vi "Drawbridge Controller.vi"(8 "error in":errorcluster) -> ()   [LabVIEW 2015]
doc: "This VI executes continuously carrying out the current operation and responding to updates or new operations. It will often contain the timing or control code that is difficult to place directly in TeleOp. This VI generally opens all sensors and motors and isolates the rest of the robot code from knowing how the operations are carried out."
uses:
  Drawbridge Setpoints.ctl
  Drawbridge Operations.ctl
  Framework/Motor Ref Names Type Def.ctl
panel:
  out "Current\nCmd":string
  # "Tip: It may be helpful to observe inputs and sensor values.\nYou may also want to display tuning or debugging controls."
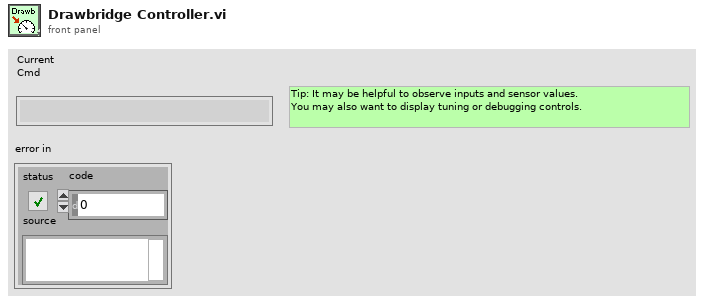
[diagram p1: front panel]
types:
  T1 = typedef "Motor Ref Names Type Def.ctl" = enum16{"Angular Motor"}
  T2 = typedef "Drawbridge Setpoints.ctl" = cluster{"Operation":T3, "Setpoint":dbl, "Duration":dbl}
  T3 = typedef "Drawbridge Operations.ctl" = enum16{"Reserve", "Read Current", "Immediate", "Open"}
  T4 = typedef "Command Status Info.ctl" = cluster{"Name":string, "Status":T5, "notifier out":T6}
  T5 = typedef "Completion Status.ctl" = enum16{"Successful", "Aborted", "Incomplete"}
  T6 = typedef "Completion Notifier.ctl" = refnum<notifier>
  T7 = cluster{"Default Command":T2, "Command Timing":cluster{"Start Time (ms)":u32, "Iterations":i32}, "Command Arguments":cluster{"Command Info":T4, "Description":string, "Default Command":T2, "notifier out":refnum<notifier>, "Subsystem Name":string}}
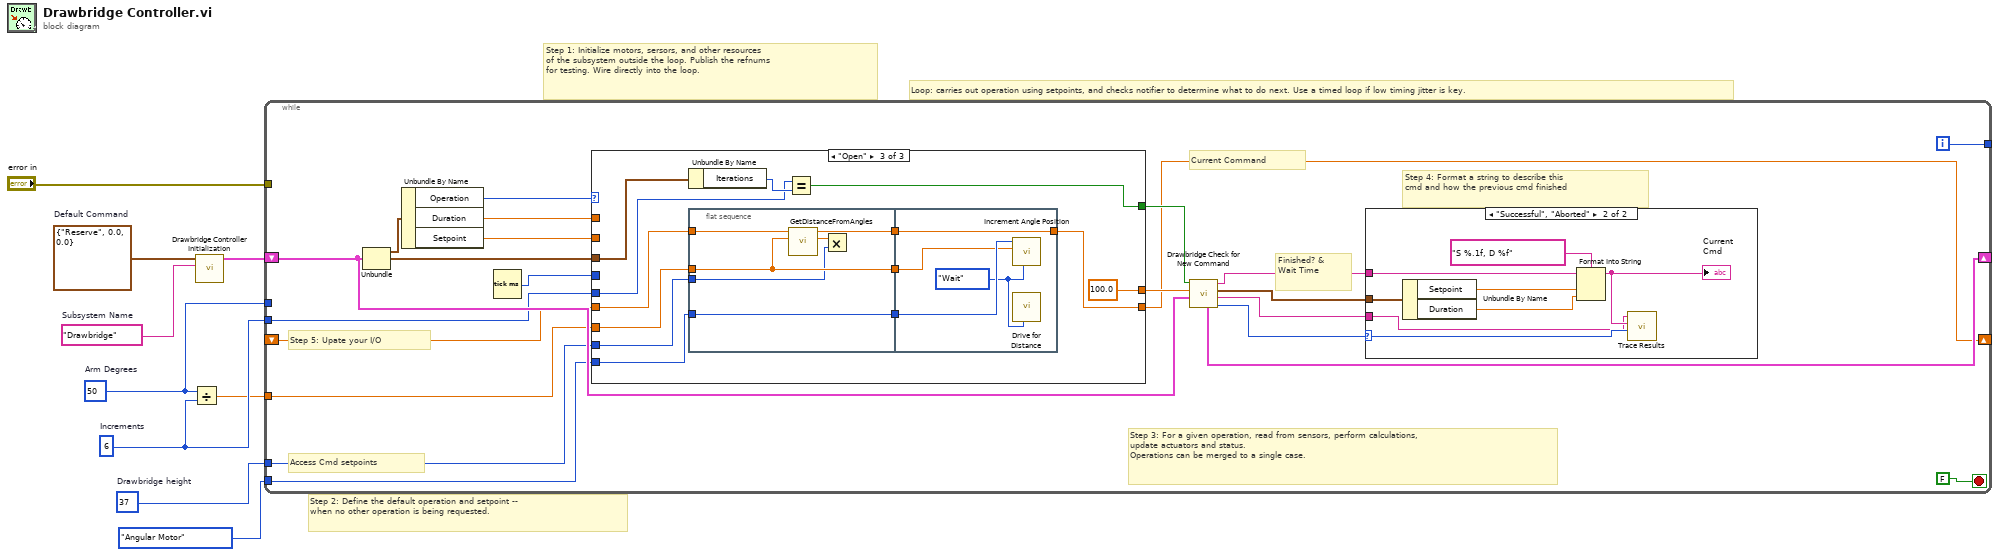
[diagram p0: block diagram]
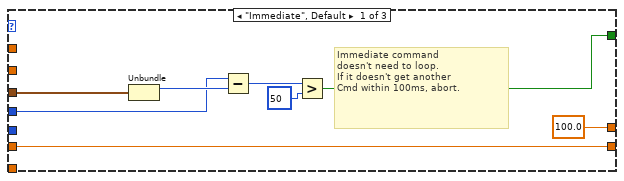
[diagram p3: hidden frame]
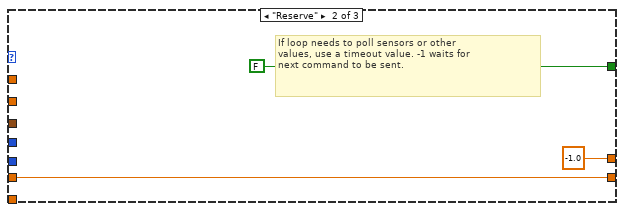
[diagram p4: hidden frame]
diagram:
  w1 = 37  # Drawbridge height
  w4 = 50  # Arm Degrees
  w3 = 6  # Increments
  w6 = T2 {"Operation"=enum."Reserve", "Setpoint"=0.0, "Duration"=0.0}  # Default Command
  w7 = "Drawbridge"  # Subsystem Name
  # "Step 2: Define the default operation and setpoint --\nwhen no other operation is being requested."
  # "Step 1: Initialize motors, sersors, and other resources\nof the subsystem outside the loop. Publish the refnums\nfor testing. Wire directly into the loop."
  # "Loop: carries out operation using setpoints, and checks notifier to determine what to do next. Use a timed loop if low timing jitter is key."
  n1 = Divide(x=w4, y=w3) -> (x/y=w2:dbl)
  n2 = call "Drawbridge Controller Initialization.vi"("Subsystem Name"=w7, "Default Command"=w6) -> ("Command Info"=w8:T7)  [unwired: 9 in]
  n3 = while {
    shift-right: [w22] -> _
    shift-left: w8 -> [w23]
    tunnel: [w30] -> _
    tunnel: "error in" -> [_]
    shift-right: [w14] -> _
    shift-left: _ -> [w15]
    tunnel: w3 -> [w13]
    tunnel: w4 -> [_]
    tunnel: Motor_Ref_Names_Type_Def."Angular Motor" ("Motor Ref Names") -> [w12]
    tunnel: w2 -> [w11]
    tunnel: w1 -> [w10]
    i -> [w30]
    stop <- FALSE stop-if-true
    # "Step 5: Upate your I/O"
    # "Step 4: Format a string to describe this\ncmd and how the previous cmd finished"
    # "Current Command"
    # "Access Cmd setpoints"
    # "Finished? &\nWait Time"
    # "Step 3: For a given operation, read from sensors, perform calculations,\nupdate actuators and status.\nOperations can be merged to a single case."
    n4 = Unbundle(w23) -> ("Default Command"=w29:T2, "Command Timing"=w25:cluster{"Start Time (ms)":u32, "Iterations":i32})  [unwired: 1 out]
    n5 = Unbundle By Name(w29) -> ("Operation"=w28:T3, "Duration"=w27:dbl, "Setpoint"=w24:dbl)
    n6 = Tick Count (ms)() -> (millisecond timer value=w26:u32)
    n7 = case shown="\"Open\"" w28 {
      tunnel: [100.0 -1.0 100.0] -> w20
      tunnel: [w41 FALSE ("ignore previous (F)") w55] -> w21
      tunnel: w25 -> [w43 _ w58]
      tunnel: w27 -> [_ _ _]
      tunnel: w26 -> [w42 _ _]
      tunnel: w24 -> [_ _ _]
      tunnel: w15 -> [w40 w48 w62]
      tunnel: w11 -> [_ _ w61]
      tunnel: [w40 w48 w59] -> w14
      tunnel: w13 -> [_ _ w56]
      tunnel: w12 -> [_ _ w53]
      tunnel: w10 -> [_ _ w51]
      frame "Immediate", Default {
        # "Immediate command\ndoesn't need to loop.\nIf it doesn't get another\nCmd within 100ms, abort."
        n8 = Unbundle(w43) -> ("Start Time (ms)"=w46:u32)  [unwired: 1 out]
        n9 = Subtract(x=w42, y=w46) -> (x-y=w45:u32)
        n10 = Greater?(x=w45, y=u8 50 ("Left Motor")) -> (0:w41:bool)
      }
      frame "Reserve" {
        # "If loop needs to poll sensors or other\nvalues, use a timeout value. -1 waits for\nnext command to be sent."
      }
      frame "Open" {
        n11 = Unbundle By Name(w58) -> ("Iterations"=w57:i32)
        n12 = flat-sequence {
          tunnel: w62 -> [w67]
          tunnel: w61 -> [w68]
          tunnel: [w66] -> w60
          tunnel: [w69] -> w54
          tunnel: w53 -> [w69]
          tunnel: [w68] -> w52
          tunnel: w51 -> [w64]
          tunnel: w60 -> [w73]
          tunnel: [w73] -> w59
          tunnel: w54 -> [w72]
          tunnel: w52 -> [w71]
          frame #0 {
            n13 = call "GetDistanceFromAngles.vi"("Next Point"=w68, "Current Point"=w67) -> ("Distance To Go"=w65:dbl, "New Point"=w66:dbl)  [unwired: 8 in]
            n14 = Multiply(x=w65, y=w64) -> ()  [unwired: 1 out]
          }
          frame #1 {
            w70 = enum16{"Start", "Wait"}."Wait" ("Synchronization")
            n15 = call "Increment Angle Position.vi"("Synchronization"=w70, "Angle"=w71, "Motor ID"=w72) -> ()  [unwired: 8 in, 1 out]
            n16 = call "Drive for Distance.vi"("Synchronization"=w70) -> ()  [unwired: 9 in, 2 out]
          }
        }
        n17 = Equal?(x=w56, y=w57) -> (x = y?=w55:bool)
      }
    }
    n18 = call "Drawbridge Check for New Command.vi"("Current Command"=w23, "Wait time (ms)"=w20, "Finished?"=w21) -> ("Completion"=w16:T5, "Subsystem Name"=w17:string, "Current Command"=w18:T2, "Initial Trace String"=w19:string, "NextCommand"=w22:T7)  [unwired: 4 in]
    n19 = case shown="\"Successful\", \"Aborted\"" w16 {
      selector: w16 -> [_ w39]
      tunnel: w19 -> [_ w35]
      tunnel: w18 -> [_ w36]
      tunnel: w17 -> [_ w32]
      frame "Incomplete", Default {
        # "Continuing current command"
      }
      frame "Successful", "Aborted" {
        # "Report and setup for next command"
        n20 = Unbundle By Name(w36) -> ("Setpoint"=w38:dbl, "Duration"=w33:dbl)
        n21 = Format Into String(format string="S %.1f, D %f", initial string=w35, w38, w33) -> (resulting string=w34:string)  [unwired: 1 in, 1 out]
        "Current\nCmd" <- w34
        n22 = call <vilib>:"Trace Results.vi"("Status of previous command"=w39, "Description"=w34, "Subsystem"=w32) -> ()  [unwired: 9 in]
      }
    }
  }
